vi "odczyt_Z_pliku_wav.vi"() -> ()   [LabVIEW 2018]
uses:
  <vilib>/sound2/lvsound2.llb/Sound File Read Open.vi
  <vilib>/sound2/lvsound2.llb/Sound File Read (DBL).vi
panel:
  in  "path":path
  in  "stop":bool
  out "Waveform Chart":waveform(dbl)[](graph)
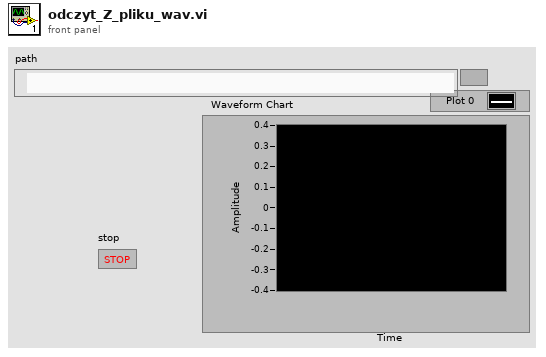
[diagram p1: front panel]
types:
  T1 = typedef "Sound File Refnum.ctl" = refnum<file>
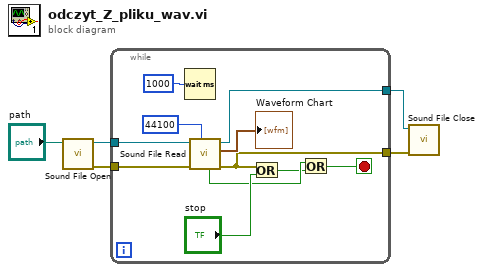
[diagram p0: block diagram]
diagram:
  n1 = call-poly <vilib>:"Sound File Open.vi"("path"="path") -> ("error out"=w4:errorcluster, "sound file refnum"=w5:T1)  [unwired: 9 in]
  n2 = while {
    tunnel: w5 -> [w15]
    tunnel: w4 -> [w7]
    tunnel: [w6] -> w3
    tunnel: [w8] -> w2
    stop <- w11 stop-if-true
    n3 = Wait (ms)(milliseconds to wait=u32 1000) -> ()  [unwired: 1 out]
    n4 = call-poly <vilib>:"Sound File Read.vi"("number of samples/ch (-1: all)"=44100, "error in (no error)"=w7, "sound file refnum"=w15) -> ("error out"=w6:errorcluster, "data"=→"Waveform Chart":waveform(dbl)[], "sound file refnum out"=w8:T1, "end of file?"=w13:bool)  [unwired: 4 in, 1 out]
    n5 = Or(x=w6, y="stop") -> (x .or. y?=w12:bool)
    n6 = Or(x=w13, y=w12) -> (x .or. y?=w11:bool)
  }
  n7 = call <vilib>:"Sound File Close.vi"("error in (no error)"=w3, "sound file refnum"=w2) -> ()  [unwired: 9 in, 1 out]
